vi "Stop Core.vi"(10 "final error code":i32, 11 "object in":refnum<class "TableLogger_SQLite_Actor.lvclass">) -> (3 "object out":refnum<class "TableLogger_SQLite_Actor.lvclass">)   [LabVIEW 2014, in "TableLogger_SQLite_Actor.lvlib" / "TableLogger_SQLite_Actor.lvclass"]
uses:
  TableLogger_SQLite_Actor.lvclass
  TableLogger_Actor/TableLogger_Actor/TableLogger_Actor.lvclass
panel:
  # "Connector Pane"
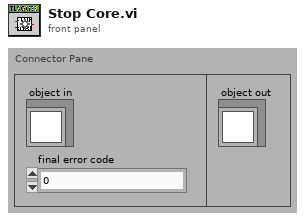
[diagram p1: front panel]
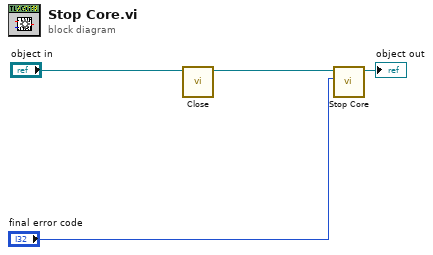
[diagram p0: block diagram]
diagram:
  n1 = call-dynamic "Close.vi"("object in"="object in") -> ("object out"=w1:refnum<class "TableLogger_SQLite_Actor.lvclass">)  [unwired: 9 in, 1 out]
  n2 = call-parent "Stop Core.vi"("final error code"="final error code", "object in"=w1) -> ("object out"=→"object out":refnum<class "TableLogger_SQLite_Actor.lvclass">)  [unwired: 9 in]
